vi "Get SMO Port.vi"(8 "error in (no error)":errorcluster, 11 "Instrument in":refnum<class "Instrument.lvclass">) -> (0 "error out":errorcluster, 2 "Port":u16, 3 "Instrument out":refnum<class "Instrument.lvclass">)   [LabVIEW 2019, in "Instrument.lvclass"]
doc: "Override this VI to return the port number of your Instrument"
uses:
  Instrument.lvclass
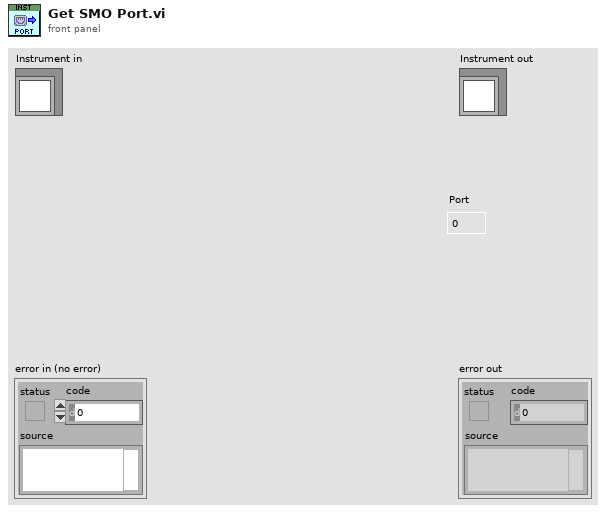
[diagram p1: front panel]
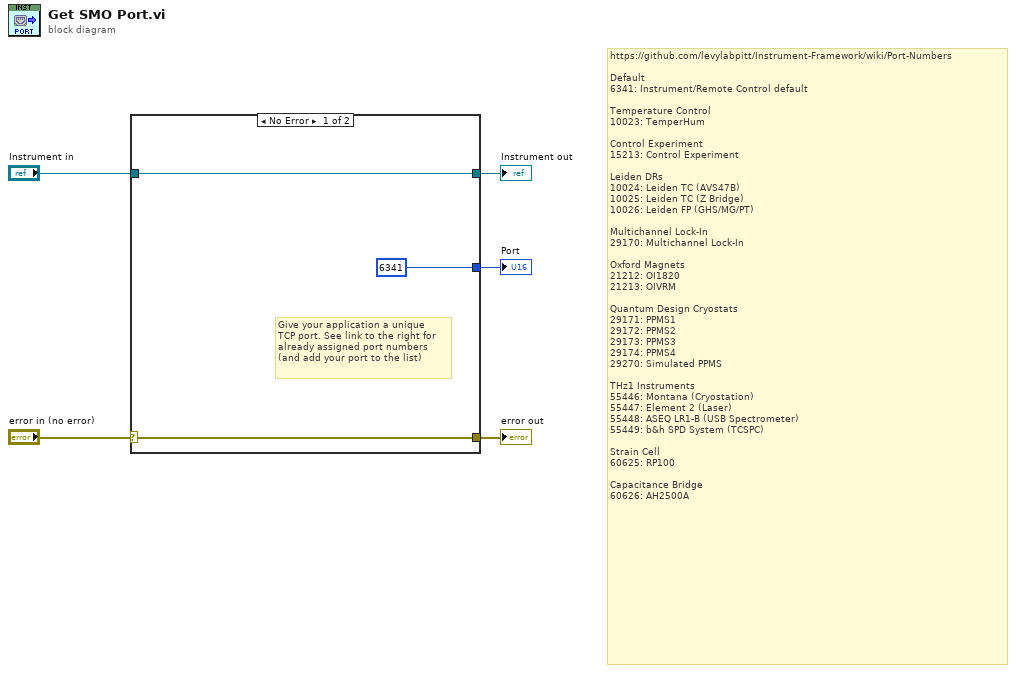
[diagram p0: block diagram]
diagram:
  # "https://github.com/levylabpitt/Instrument-Framework/wiki/Port-Numbers\n\nDefault\n6341: Instrument/Remote Control default\n\nTemperature Control\n10023: TemperHum\n\nControl Experiment\n15213: Control Experiment\n\nLeiden DRs\n10024: Leiden TC (AVS47B)\n10025: Leiden TC (Z Bridge)\n10026: Leiden FP (GHS/MG/PT)\n\nMultichannel Lock-In\n29170: Multichannel Lock-In\n\nOxford Magnets\n21212: OI1820\n21213: OIVRM\n\nQuantum Design Cryostats\n29171: PPMS1\n29172: PPMS2\n29173: PPMS3\n29174: PPMS4\n29270: Simulated PPMS\n\nTHz1 Instruments\n55446: Montana (Cryostation)\n55447: Element 2 (Laser)\n55448: ASEQ LR1-B (USB Spectrometer)\n55449: b&h SPD System (TCSPC)\n\nStrain Cell\n60625: RP100\n\nCapacitance Bridge\n60626: AH2500A"
  n1 = case shown="No Error" "error in (no error)" {
    selector: "error in (no error)" -> [w8 w10]
    tunnel: [w8 w10] -> w4
    tunnel: [w6 w9] -> w2
    tunnel: "Instrument in" -> [w6 w9]
    tunnel: [u16 6341 ("Port") _] -> w1
    frame No Error {
      # "Give your application a unique\nTCP port. See link to the right for\nalready assigned port numbers\n(and add your port to the list)"
    }
    frame Error {
    }
  }
  "error out" <- w4
  "Instrument out" <- w2
  "Port" <- w1
